vi "DriveStraightv3.vi"(4 "EncData":T1, 6 "Decel?":bool, 7 "GyroData":T2, 8 "Accel?":bool, 9 "FirstTime?":bool, 10 "MinPwr":dbl, 11 "MtrPwr":dbl) -> (0 "RightOut":dbl, 3 "LeftOut":dbl)   [LabVIEW 2017]
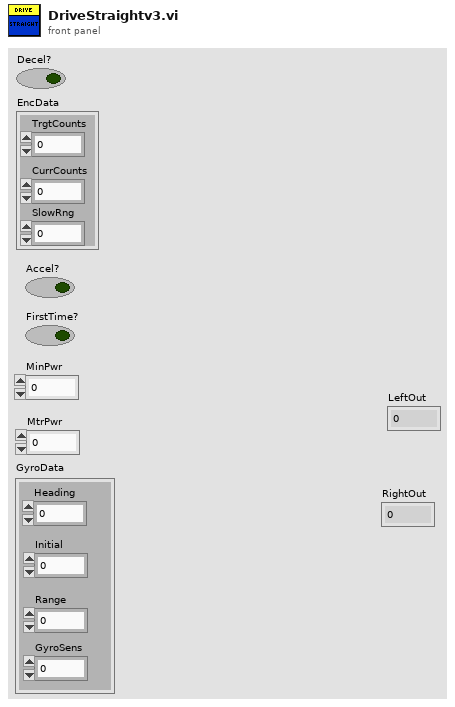
[diagram p1: front panel]
types:
  T1 = cluster{"TrgtCounts":i32, "CurrCounts":dbl, "SlowRng":dbl}
  T2 = cluster{"Heading":dbl, "Initial":dbl, "Range":dbl, "GyroSens":dbl}
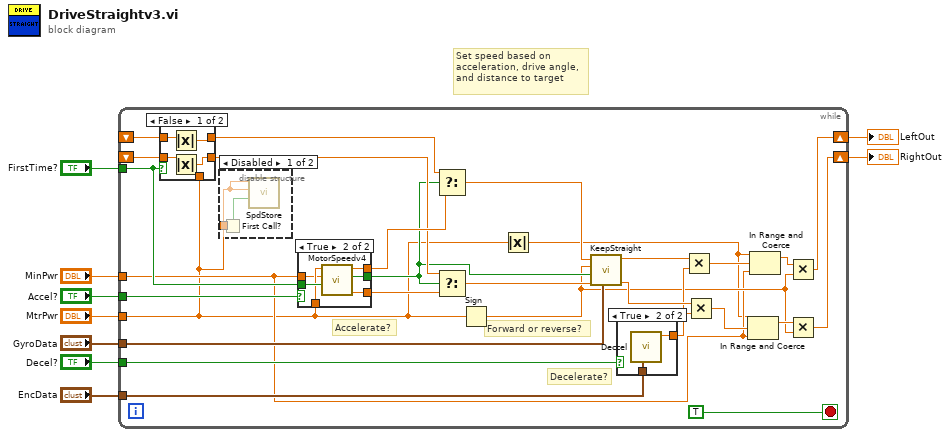
[diagram p0: block diagram]
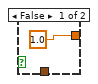
[diagram p4: hidden frame]
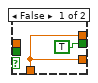
[diagram p5: hidden frame]
diagram:
  # "Set speed based on\nacceleration, drive angle,\nand distance to target"
  n1 = while {
    tunnel: "MtrPwr" -> [w11]
    tunnel: "FirstTime?" -> [w25]
    shift-right: [w13] -> w8
    shift-left: _ -> [w26]
    shift-right: [w14] -> w7
    shift-left: _ -> [w29]
    tunnel: "MinPwr" -> [w12]
    tunnel: "Accel?" -> [w36]
    tunnel: "GyroData" -> [w24]
    tunnel: "Decel?" -> [w31]
    tunnel: "EncData" -> [w30]
    stop <- TRUE stop-if-true
    # "Decelerate?"
    # "Accelerate?"
    # "Forward or reverse?"
    n2 = case shown="False" w25 {
      tunnel: w29 -> [w43 _]
      tunnel: [w40 w44] -> w28
      tunnel: [w41 w44] -> w27
      tunnel: w26 -> [w42 _]
      tunnel: w11 -> [_ w44]
      frame False {
        n3 = Absolute Value(x=w43) -> (abs(x)=w40:dbl)
        n4 = Absolute Value(x=w42) -> (abs(x)=w41:dbl)
        n5 = Absolute Value(x=w42) -> ()  [unwired: 1 out]
      }
      frame True {
      }
    }
    n6 = disable-structure shown="Disabled" {
      disable-tunnel: w11 -> [w39 _]
      frame Disabled {
        n7 = First Call?() -> (First Call?: T/F=w38:bool)
        n8 = call "SpdStore.vi"("Update?"=w38, "RightSpdIn"=w39, "LeftSpdIn"=w39) -> ()  [unwired: 7 in, 2 out]
      }
      frame Enabled {
      }
    }
    n9 = case shown="True" w36 {
      tunnel: [w48 w55] -> w35
      tunnel: [w48 w54] -> w34
      tunnel: [TRUE ("Acceled?") w53] -> w23
      tunnel: w25 -> [_ w52]
      tunnel: w11 -> [w48 w51]
      tunnel: w12 -> [_ w50]
      frame False {
      }
      frame True {
        n10 = call "MotorSpeedv4.vi"("FirstTime?"=w52, "MinPwr"=w50, "MaxPwr"=w51) -> ("RightSpdOut"=w54:dbl, "Acceled?"=w53:bool, "LeftSpdOut"=w55:dbl)  [unwired: 6 in]
      }
    }
    n11 = Select(t=w28, s=w23, f=w35) -> (s? t:f=w33:dbl)
    n12 = Select(t=w27, s=w23, f=w34) -> (s? t:f=w32:dbl)
    n13 = Sign(1:w11) -> (0:w15:dbl)
    n14 = Absolute Value(x=w11) -> (abs(x)=w10:dbl)
    n15 = call "KeepStraight.vi"("GyroData"=w24, "RightSpdIn"=w32, "AccelDone?"=w23, "MtrDir"=w15, "LeftSpdIn"=w33) -> ("RightSpdOut"=w21:dbl, "LeftSpdOut"=w22:dbl)  [unwired: 5 in]
    n16 = case shown="True" w31 {
      tunnel: [1.0 ("SpdMult") w47] -> w20
      tunnel: w30 -> [_ w46]
      frame False {
      }
      frame True {
        n17 = call "Deccel.vi"("EncData"=w46) -> ("SpdMult"=w47:dbl)  [unwired: 10 in]
      }
    }
    n18 = Multiply(x=w22, y=w20) -> (x*y=w19:dbl)
    n19 = Multiply(x=w21, y=w20) -> (x*y=w18:dbl)
    n20 = In Range and Coerce(upper limit=w10, x=w18, lower limit=w12) -> (coerced(x)=w16:dbl)  [unwired: 1 out]
    n21 = In Range and Coerce(upper limit=w10, x=w19, lower limit=w12) -> (coerced(x)=w17:dbl)  [unwired: 1 out]
    n22 = Multiply(x=w17, y=w15) -> (x*y=w14:dbl)
    n23 = Multiply(x=w16, y=w15) -> (x*y=w13:dbl)
  }
  "LeftOut" <- w7
  "RightOut" <- w8
